vi "Delete Bucket.vi"(8 "error in (no error)":errorcluster, 11 "Bucket":refnum<class "Bucket.lvclass">) -> (0 "error out":errorcluster)   [LabVIEW 2015, in "NI_AWS_S3.lvlib" / "Bucket.lvclass"]
doc: "This implementation of the DELETE operation deletes the bucket named in the URI. All objects (including all object versions and delete markers) in the bucket must be deleted before the bucket itself can be deleted."
uses:
  Bucket.lvclass
  Core/HTTP Request/Region handling.ctl
  Core/HTTP Request/Request Options.ctl
  Core/HTTP Request/Name Value Pair.ctl
  Core/HTTP Request/URL formatting.ctl
  Bucket.lvclass/Bucket.ctl
  Read Name.vi
  Core/HTTP Request/HTTP Request.lvclass
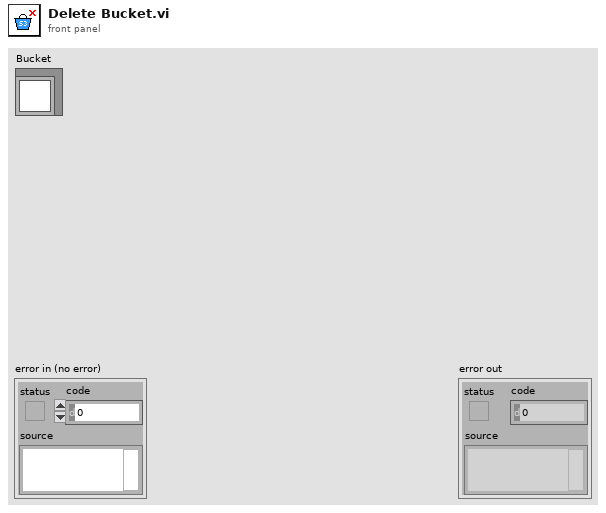
[diagram p1: front panel]
types:
  T1 = typedef "NI_AWS_Core.lvlib/HTTP Request.lvclass/Request Options.ctl" = cluster{"request headers":T2[], "request parameters":T2[], "request body":string, "region handling":T3, "URL formatting":T4}
  T2 = typedef "NI_AWS_Core.lvlib/HTTP Request.lvclass/Name Value Pair.ctl" = cluster{"name":string, "value":string}
  T3 = typedef "NI_AWS_Core.lvlib/HTTP Request.lvclass/Region handling.ctl" = enum16{"use region everywhere", "use region (authentication only)", "use region (URL only)", "ignore region everwhere"}
  T4 = typedef "NI_AWS_Core.lvlib/HTTP Request.lvclass/URL formatting.ctl" = enum16{"region-", "region."}
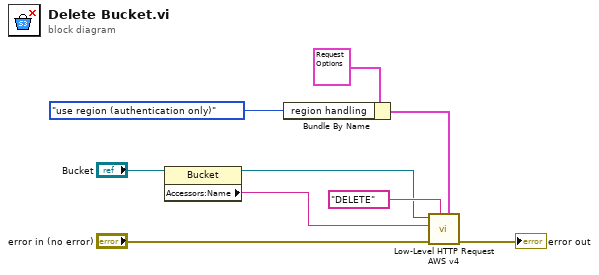
[diagram p0: block diagram]
diagram:
  n1 = property class="Bucket"(reference="Bucket") -> (reference out=w1:refnum<class "Bucket.lvclass">, "Accessors:Name"=w6:string)  [unwired: 1 in, 1 out]
  n2 = Bundle By Name(cluster=T1 {"request headers"=[], "request parameters"=[], "request body"="", "region handling"=enum."use region everywhere", "URL formatting"=enum."region."} ("Request Options"), "region handling"=Region_handling."use region (authentication only)") -> (w3:T1)
  n3 = call "Low-Level HTTP Request AWS v4.vi"("Request Options"=w3, "HTTP-Verb"="DELETE", "error in (no error)"="error in (no error)", "URL Prefix"=w6, "AWS Core in"=w1) -> ("error out"=→"error out":errorcluster)  [unwired: 3 in, 3 out]
